vi "Set Minimum Panel Size.vi"(8 "error in (no error)":errorcluster, 10 "Minimum Size":T1, 11 "IViewable In":refnum<class "IViewable.lvclass">) -> (0 "error out":errorcluster, 3 "IViewable Out":refnum<class "IViewable.lvclass">)   [LabVIEW 2017, in "IViewable.lvlib" / "IViewable.lvclass"]
doc: "<License>\nCopyright © 2017 Composed Systems, LLC | All rights reserved\nwww.composed.io\n\nAuthor: Ethan Stern <ethan.stern@composed.io>\n\nThis software is provided \"AS IS\" WITHOUT WARRANTIES, either express or implied, AND IS FOR EDUCATIONAL PURPOSES ONLY.\n</License>"
uses:
  IViewable.lvclass
  <vilib>/Utility/miscctls.llb/LVPointTypeDef.ctl
  IViewable.lvclass/IViewable.ctl
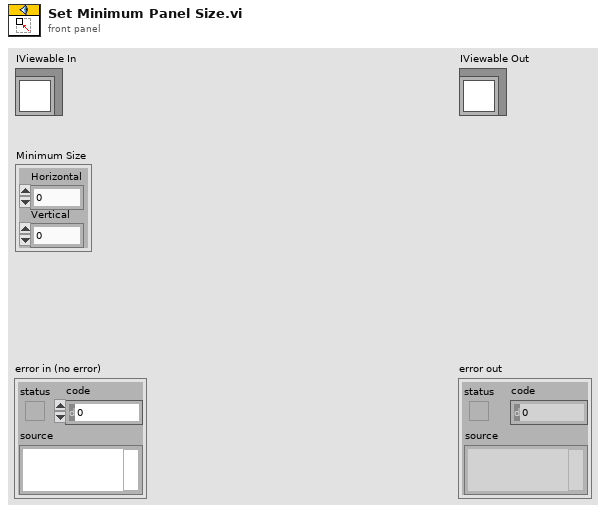
[diagram p1: front panel]
types:
  T1 = typedef "LVPointTypeDef.ctl" = cluster{"Horizontal":i16, "Vertical":i16}
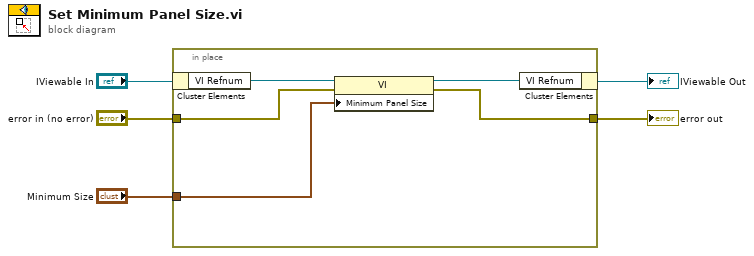
[diagram p0: block diagram]
diagram:
  n1 = in-place {
    in-place-border: "Minimum Size" -> [w8]
    in-place-border: "error in (no error)" -> [w7]
    in-place-border: [w6] -> w1
    n2 = in-place-cluster #1("IViewable In") -> ("VI Refnum"=w10:refnum<vi>)
    n3 = property class="VI"(reference=w10, error in=w7, "Minimum Panel Size"=w8) -> (reference out=w9:refnum<vi>, error out=w6:errorcluster)
    n4 = in-place-cluster #1("VI Refnum"=w9) -> (→"IViewable Out":refnum<class "IViewable.lvclass">)
  }
  "error out" <- w1
